vi "sin(x).vi"() -> ()   [LabVIEW 2023]
panel:
  in  "x":dbl=1.0 format="%#_13g"
  out "Waveform Graph":dbl[][](graph)
  out "Waveform Chart":dbl(graph)
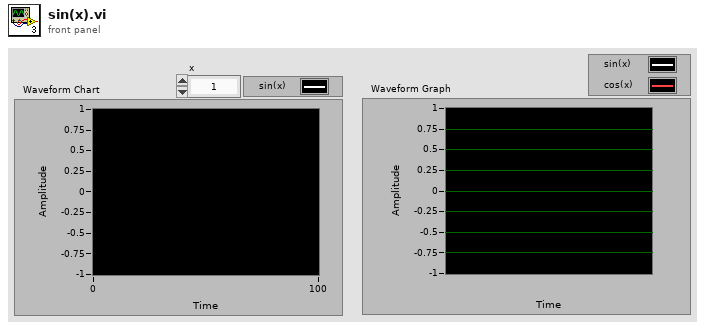
[diagram p1: front panel]
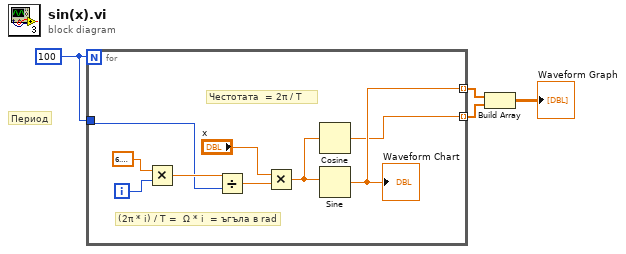
[diagram p0: block diagram]
diagram:
  w4 = 100
  # "Период"
  n1 = for {
    N: w4 -> [_]
    tunnel: w4 -> [w10]
    tunnel: [w7] -> w3 mode=indexing
    tunnel: [w5] -> w1 mode=indexing
    i -> [w13]
    # "(2π * i) / T =  Ω * i  = ъгъла в rad"
    # "Честотата  = 2π / T"
    n2 = Multiply(x=6.283185307179586, y=w13) -> (x*y=w11:dbl)
    n3 = Divide(x=w11, y=w10) -> (x/y=w9:dbl)
    n4 = Multiply(x="x", y=w9) -> (x*y=w6:dbl)
    n5 = Cosine(x=w6) -> (cos(x)=w5:dbl)
    n6 = Sine(x=w6) -> (sin(x)=w7:dbl)
    "Waveform Chart" <- w7
  }
  n7 = Build Array(w3, w1) -> (→"Waveform Graph":dbl[][])
